vi "SVL Exp Avg Level (N Ch).vi"(6 "restart averaging (F)":bool, 8 "error in (no error)":errorcluster, 9 "time constant [ms]":dbl=125.0 format="%.2f", 10 "exponential mode":enum16{"Slow", "Fast", "Impulse", "Custom"}(ring)=enum."Fast", 11 "scaled signals [EU]":waveform(dbl)[](array[waveform])) -> (0 "error out":errorcluster, 1 "actual time constant [ms]":dbl=nan format="%.2f", 2 "unit labels":string[](array[string]), 3 "exp avg levels [EU rms]":waveform(dbl)[](array[waveform]))   [LabVIEW 2017, in "SoundVib_VibrationLevel.lvlib"]
doc: "Computes the exponential averaged level of <B>scaled signal [EU]</B> or <B>even-angle signal [EU]</B>. <B>scaled signal [EU]</B> should have a zero DC component. You can attenuate the DC component with hardware AC-coupling filters and with software high-pass filters. Wire data to the <B>scaled signal [EU]</B> input to determine the polymorphic instance to use or manually select the instance."
uses:
  <vilib>/addons/Sound and Vibration/svt_Level/SoundVib_VibrationLevel.lvlib
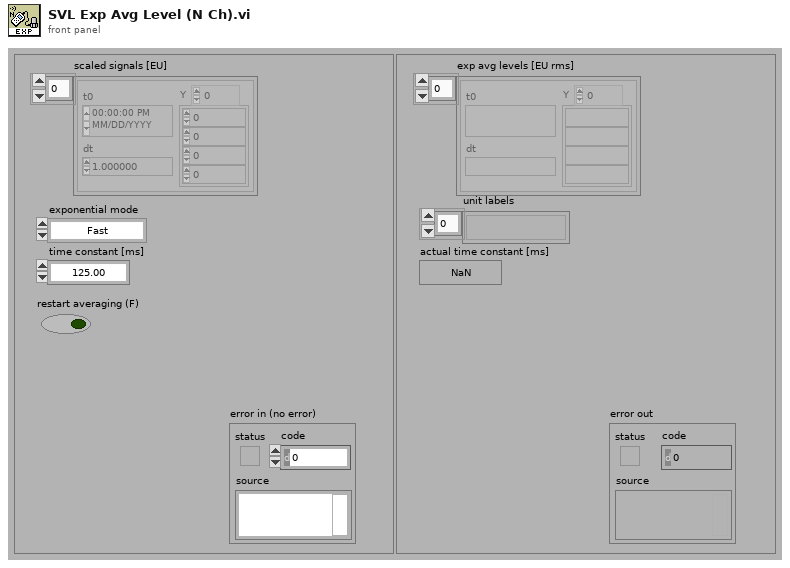
[diagram p1: front panel]
types:
  T1 = enum16{"RMS", "Running RMS", "Exp avg  ", "Dec exp avg ", "Peak", "Crest"}
  T2 = enum16{"Reset filter", "Restart averaging", "Continue processing"}
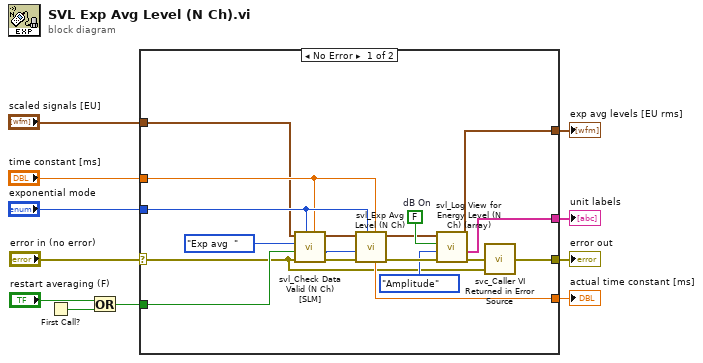
[diagram p0: block diagram]
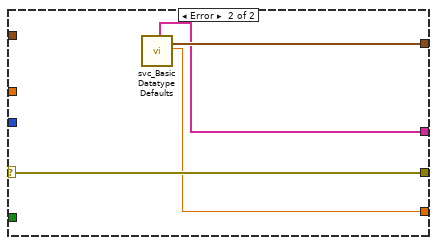
[diagram p2: hidden frame]
diagram:
  n1 = First Call?() -> (First Call?: T/F=w10:bool)
  n2 = Or(x="restart averaging (F)", y=w10) -> (x .or. y?=w9:bool)
  n3 = case shown="No Error" "error in (no error)" {
    selector: "error in (no error)" -> [w12 w33]
    tunnel: w9 -> [w18 _]
    tunnel: "scaled signals [EU]" -> [w16 _]
    tunnel: [w13 w32] -> w7
    tunnel: [w19 w33] -> w6
    tunnel: [w24 w31] -> w5
    tunnel: "exponential mode" -> [w23 _]
    tunnel: "time constant [ms]" -> [w22 _]
    tunnel: [w20 w30] -> w2
    frame No Error {
      w27 = FALSE  # dB On
      n4 = call <vilib>:"svl_Check Data Valid (N Ch) [SLM].vi"("time constant [ms]"=w22, "exponential mode"=w23, "error in (no error)"=w12, "restart averaging (F)"=w18, "level analysis"=T1."Exp avg  " ("Level Analysis"), "scaled signals [EU]"=w16) -> ("error out"=w29:errorcluster, "processing state"=w21:T2, "dup scaled signals [EU]"=w15:waveform(dbl)[])  [unwired: 3 in]
      n5 = call <vilib>:"svl_Exp Avg Level (N Ch).vi"("timeConstant"=w22, "exponential mode"=w23, "error in (no error)"=w29, "processing state"=w21, "scaled signals"=w15) -> ("error out"=w28:errorcluster, "exp avg signals"=w14:waveform(dbl)[], "actual time constant [ms]"=w20:dbl)  [unwired: 3 in, 1 out]
      n6 = call <vilib>:"svl_Log View for Energy Level (N Ch) (array).vi"("error in (no error)"=w28, "view mode"=enum16{"Power", "Amplitude"}."Amplitude", "dB On (T)"=w27, "scaled signals"=w14) -> ("error out"=w25:errorcluster, "unit labels"=w24:string[], "scaled signals"=w13:waveform(dbl)[])  [unwired: 5 in]
      n7 = call <vilib>:"svc_Caller VI Returned in Error Source.vi"("warning input to caller"=w12, "error in (no error)"=w25) -> ("error out"=w19:errorcluster)  [unwired: 3 in]
    }
    frame Error {
      n8 = call <vilib>:"svc_Basic Datatype Defaults.vi"() -> ("empty array of strings"=w31:string[], "empty array of waveforms"=w32:waveform(dbl)[], "NaN"=w30:dbl)  [unwired: 7 in, 10 out]
    }
  }
  "exp avg levels [EU rms]" <- w7
  "actual time constant [ms]" <- w2
  "unit labels" <- w5
  "error out" <- w6
